vi "Preview Message.vi"(8 "error in (no error)":errorcluster, 10 "timeout in ms (-1)":i32=-1, 11 "Message Queue":refnum<queue>) -> (0 "error out":errorcluster, 1 "Message Data":variant, 2 "Message":string, 3 "dup Message Queue":refnum<queue>, 4 "timed out?":bool)   [LabVIEW 2014, in "Message Queue.lvlib"]
doc: "This VI pulls messages off the Message Queue."
uses:
  Message Queue.lvlib
  Message Cluster.ctl
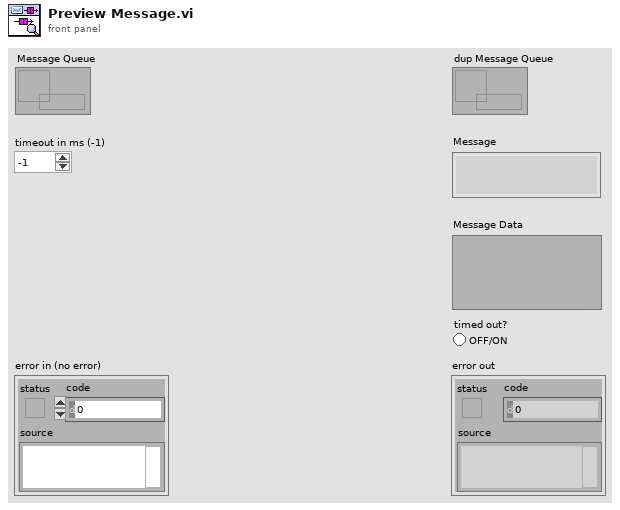
[diagram p1: front panel]
types:
  T1 = typedef "Message Queue.lvlib/Message Cluster.ctl" = cluster{"Message":string, "Message Data":variant}
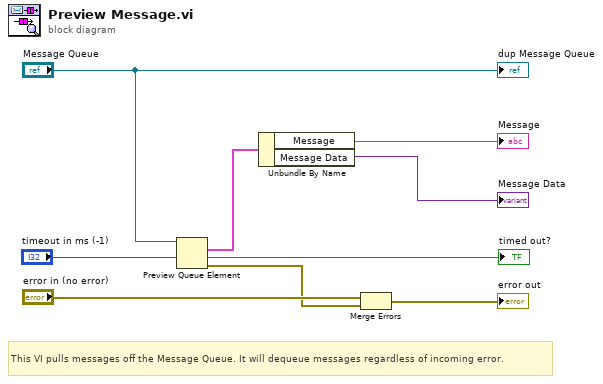
[diagram p0: block diagram]
diagram:
  # "This VI pulls messages off the Message Queue. It will dequeue messages regardless of incoming error."
  n1 = Preview Queue Element(queue="Message Queue", timeout in ms (-1)="timeout in ms (-1)") -> (element=w6:T1, timed out?=→"timed out?":bool, error out=w3:errorcluster)  [unwired: 1 in, 1 out]
  n2 = Unbundle By Name(w6) -> ("Message"=→"Message":string, "Message Data"=→"Message Data":variant)
  n3 = Merge Errors("error in (no error)", w3) -> (→"error out":errorcluster)
  "dup Message Queue" <- "Message Queue"
